vi "Destructor.vi"(8 "error in":errorcluster, 11 "SequenceRun":refnum<class "SequenceRun.lvclass">) -> (0 "error out":errorcluster)   [LabVIEW 2021, in "ProligentXMLGenerator.lvlib" / "SequenceRun.lvclass"]
uses:
  SequenceRun.lvclass
  SequenceRun.lvclass/SequenceRun.ctl
  StepRun/StepRun/StepRun.lvclass
  Model/CustomData/CustomData.lvclass
  Model/Characteristic/Characteristic.lvclass
  Model/Document/Document.lvclass
  Failure/FailureReference/FailureReference.lvclass
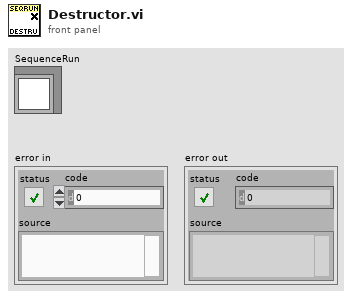
[diagram p1: front panel]
types:
  T1 = typedef "ProligentXMLGenerator.lvlib/SequenceRun.lvclass/Data.ctl" = cluster{"Name":string, "StepRuns":refnum<class "StepRun.lvclass">[], "Characteristics":refnum<class "Characteristic.lvclass">[], "Documents":refnum<class "Document.lvclass">[], "FailureReferences":refnum<class "FailureReference.lvclass">[], "CustomData":refnum<class "CustomData.lvclass">, "StartDate":refnum<class "DateTime.lvclass">, "EndDate":refnum<class "DateTime.lvclass">, "SequenceExecutionStatus":refnum<class "ExecutionStatus.lvclass">, "SequenceRunId":refnum<class "Guid.lvclass">, "SequenceFullName":refnum<class "SequenceFullName.lvclass">, "SequenceVersion":refnum<class "NonEmptyString_64.lvclass">, "StationFullName":refnum<class "FullName.lvclass">, "User":refnum<class "NonEmptyString_255.lvclass">, "TimeZoneInfoId":string}
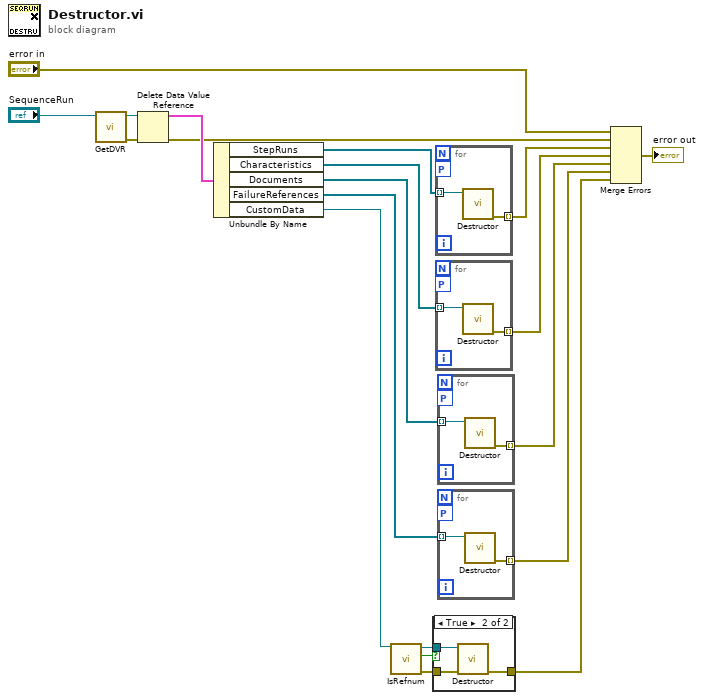
[diagram p0: block diagram]
diagram:
  n1 = call "GetDVR.vi"("SequenceRun"="SequenceRun") -> ("error out"=w17:errorcluster, "DVRReference"=w18:refnum<data-value>)  [unwired: 9 in]
  n2 = Delete Data Value Reference(data value reference=w18, error in=w17) -> (data value=w16:T1, error out=w12:errorcluster)
  n3 = Unbundle By Name(w16) -> ("StepRuns"=w13:refnum<class "StepRun.lvclass">[], "Characteristics"=w11:refnum<class "Characteristic.lvclass">[], "Documents"=w10:refnum<class "Document.lvclass">[], "FailureReferences"=w9:refnum<class "FailureReference.lvclass">[], "CustomData"=w5:refnum<class "CustomData.lvclass">)
  n4 = call "IsRefnum.vi"("CustomDataType in"=w5) -> ("error out"=w8:errorcluster, "IsRefnum"=w7:bool, "CustomDataType out"=w6:refnum<class "CustomData.lvclass">)  [unwired: 8 in]
  n5 = case shown="True" w7 {
    tunnel: w8 -> [w21 w24]
    tunnel: [w21 w23] -> w1
    tunnel: w6 -> [_ w22]
    frame False {
    }
    frame True {
      n6 = call "Destructor.vi"("error in"=w24, "CustomDataType"=w22) -> ("error out"=w23:errorcluster)  [unwired: 9 in]
    }
  }
  n7 = for {
    tunnel: w13 -> [w26] mode=indexing
    tunnel: [w25] -> w14 mode=indexing
    workers-P: _ -> [_]
    n8 = call "Destructor.vi"("StepRun"=w26) -> ("error out"=w25:errorcluster)  [unwired: 10 in]
  }
  n9 = for {
    tunnel: w11 -> [w28] mode=indexing
    tunnel: [w27] -> w4 mode=indexing
    workers-P: _ -> [_]
    n10 = call "Destructor.vi"("Document in"=w28) -> ("error out"=w27:errorcluster)  [unwired: 10 in]
  }
  n11 = for {
    tunnel: w10 -> [w30] mode=indexing
    tunnel: [w29] -> w3 mode=indexing
    workers-P: _ -> [_]
    n12 = call "Destructor.vi"("Document in"=w30) -> ("error out"=w29:errorcluster)  [unwired: 10 in]
  }
  n13 = for {
    tunnel: w9 -> [w32] mode=indexing
    tunnel: [w31] -> w2 mode=indexing
    workers-P: _ -> [_]
    n14 = call "Destructor.vi"("FailureReference in"=w32) -> ("error out"=w31:errorcluster)  [unwired: 10 in]
  }
  n15 = Merge Errors("error in", w12, w14, w4, w3, w2, w1) -> (→"error out":errorcluster)
